vi "图像对称、曲面操作2.vi"() -> ()   [LabVIEW 2018]
uses:
  <vilib>/vision/NI_Vision_Development_Module.lvlib
panel:
  out "Image 4":T1(plugin-control)
  out "Image 3":T1(plugin-control)
  out "error out":errorcluster
  out "Image 2":T1(plugin-control)
  out "Image":T1(plugin-control)
  in  "路径":path
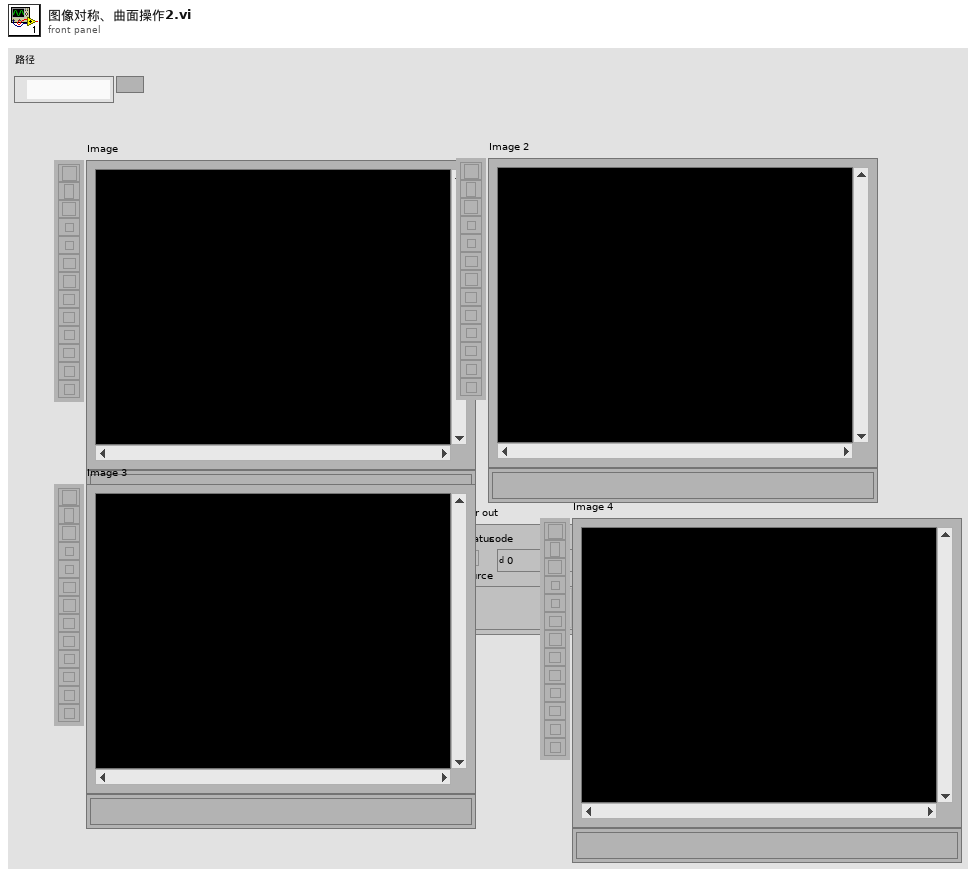
[diagram p1: front panel]
types:
  T1 = typedef "IMAQ Image.ctl" = refnum<image>
  T2 = typedef "IMAQ Circle" = cluster{"Center X":i32, "Center Y":i32, "Inner Radius":i32, "Outer Radius":i32, "Start Angle":dbl, "End Angle":dbl}
  T3 = typedef "ROI Descriptor" = cluster{"Global Rectangle":i32[], "Contours":cluster{"ID":enum32{"External", "Internal"}, "Type":u32, "Coordinates":i32[]}[]}
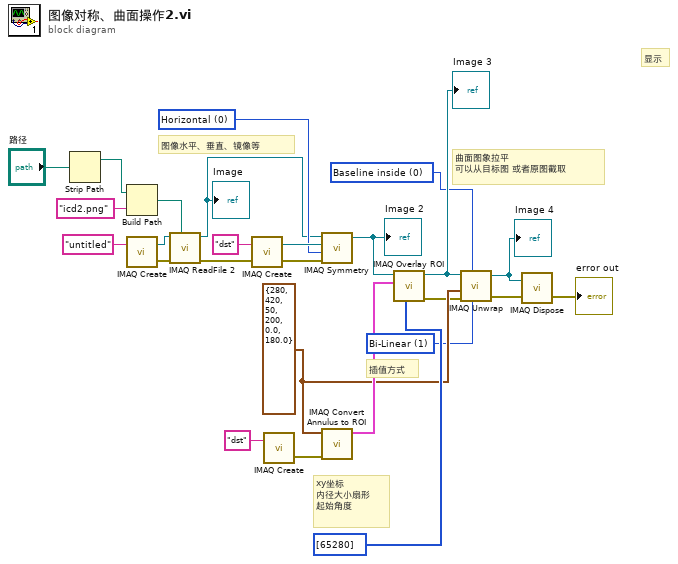
[diagram p0: block diagram]
diagram:
  w1 = u32 0 items=["Baseline inside", "Baseline outside"] ("Orientation")
  w4 = u32 1 items=["Zero Order", "Bi-Linear", "Quadratic", "Cubic Spline"] ("Interpolation Type")
  w7 = T2 {"Center X"=280, "Center Y"=420, "Inner Radius"=50, "Outer Radius"=200, "Start Angle"=0.0, "End Angle"=180.0} ("Annulus")
  w16 = u32 0 items=["Horizontal", "Vertical", "Central", "1st Diagonal", "2nd Diagonal"] ("Type of Symmetry")
  # "插值方式"
  # "显示"
  # "xy坐标\n内径大小扇形\n起始角度"
  # "曲面图象拉平\n可以从目标图 或者原图截取"
  # "图像水平、垂直、镜像等"
  n1 = Strip Path(path="路径") -> (stripped path=w25:path)  [unwired: 1 out]
  n2 = Build Path(base path=w25, name or relative path="icd2.png" ("名称或相对路径")) -> (appended path=w14:path)
  n3 = call "IMAQ Create"("Image Name"="untitled") -> ("New Image"=w23:T1, "error out"=w22:errorcluster)  [unwired: 4 in]
  n4 = call "IMAQ ReadFile 2"("File Path"=w14, "error in (no error)"=w22, "Image"=w23) -> ("error out"=w20:errorcluster, "Image Out"=w15:T1)  [unwired: 4 in, 3 out]
  "Image" <- w15
  n5 = call "IMAQ Create"("Image Name"="dst", "error in (no error)"=w20) -> ("New Image"=w18:T1, "error out"=w17:errorcluster)  [unwired: 3 in]
  n6 = call "IMAQ Create"("Image Name"="dst") -> ("error out"=w11:errorcluster)  [unwired: 4 in, 1 out]
  n7 = call "IMAQ Symmetry"("error in (no error)"=w17, "Type of Symmetry"=w16, "Image Dst"=w18, "Image Src"=w15) -> ("Image Dst Out"=w10:T1)  [unwired: 1 in, 1 out]
  "Image 2" <- w10
  n8 = call "IMAQ Convert Annulus to ROI"("error in (no error)"=w11, "Annulus"=w7) -> ("ROI Descriptor"=w9:T3)  [unwired: 7 in, 1 out]
  n9 = call "IMAQ Overlay ROI"("Colors (Green)"=u32[] [65280], "ROI Descriptor"=w9, "Image"=w10) -> ("error out"=w5:errorcluster, "Image Out"=w6:T1)  [unwired: 7 in]
  "Image 3" <- w6
  n10 = call "IMAQ Unwrap"("Image Src"=w6, "Orientation"=w1, "Annulus"=w7, "Interpolation Type"=w4, "error in (no error)"=w5) -> ("Image Dst Out"=w2:T1, "error out"=w3:errorcluster)  [unwired: 2 in]
  "Image 4" <- w2
  n11 = call "IMAQ Dispose"("Image"=w2, "error in (no error)"=w3) -> ("error out"=→"error out":errorcluster)  [unwired: 4 in]
